vi "c ctre phoenixpro deserialize int.vi"(7 "val":i32, 8 "error in (no error)":errorcluster, 9 "strlen":u32, 10 "str":string, 11 "spn":i32) -> (0 "error out":errorcluster, 3 "function return":i32, 5 "val out":i32)   [LabVIEW 2020, in "CTRE_PhoenixTools.lvlib"]
doc: "CTREXPORT int c_ctre_phoenixpro_deserialize_int(int spn, const char *str, uint32_t strlen, int *val);"
uses:
  CTRE_PhoenixTools.lvlib
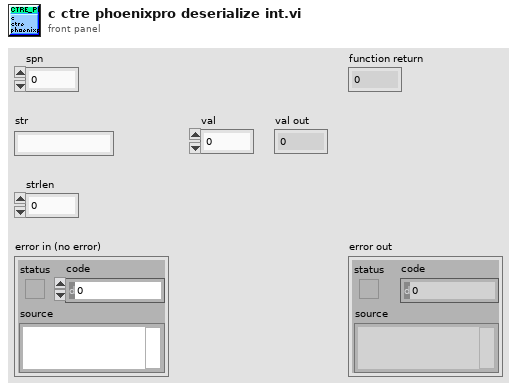
[diagram p1: front panel]
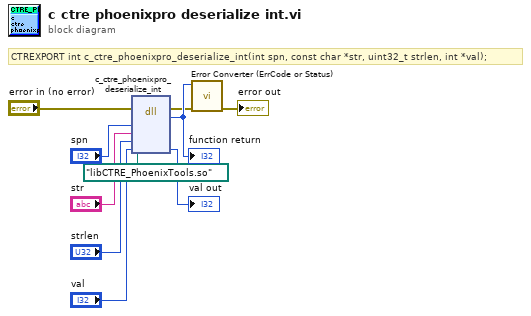
[diagram p0: block diagram]
diagram:
  # "CTREXPORT int c_ctre_phoenixpro_deserialize_int(int spn, const char *str, uint32_t strlen, int *val);"
  n1 = dll-call lib="?" fn="c_ctre_phoenixpro_deserialize_int"(path in=path "libCTRE_PhoenixTools.so", error in="error in (no error)", "spn"="spn", "str"="str", "strlen"="strlen", "val"="val") -> (error out=w3:errorcluster, w10:i32, "val"=→"val out":i32)  [unwired: 4 in, 1 out]
  "function return" <- w10
  n2 = call "Error Converter (ErrCode or Status).vi"("error in (no error)"=w3, "error code"=w10) -> ("error out"=→"error out":errorcluster)  [unwired: 9 in]
